vi "Keithley 2200 Series Execute a List.vi"() -> ()   [LabVIEW 2021]
doc: "DESCRIPTION:\n\nIn this VI commands executed in a certain order to run the list file. \n\nINSTRUCTIONS:\n1. Enter the resource name.\n2. Configures the power supply for command List mode\n3. Recall operation , recall list file from memory \n4. Enter Non -volatile memory address, that the settings will be saved to. \n5. Enable output of the power supply.\n6. Set trigger command to run the list file.\n7. Run the VI.\n\nNOTES:\n\nNotice the order of the power supply component VIs in the block diagram. The first VI in a sequence is the power supply Initialize.vi, which provides a VISA session to the instrument driver. The last VI in a sequence must be the power supply Close.vi which closes the Visa session."
uses:
  <instrlib>/Keithley 2200 Series/Keithley 2200 Series.lvlib
panel:
  in  "Enable Output (T: Enable)":bool=TRUE
  in  "VISA resource name":refnum<visa-resource-name>
  in  "Memory Address(1)":dbl=1.0
  # "(c) Copyright 2012 Keithley Instruments Inc  ALL RIGHTS RESERVED."
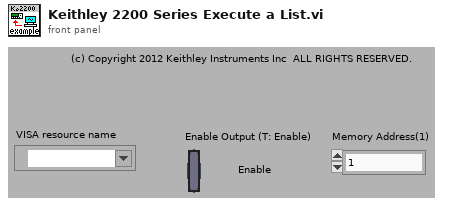
[diagram p1: front panel]
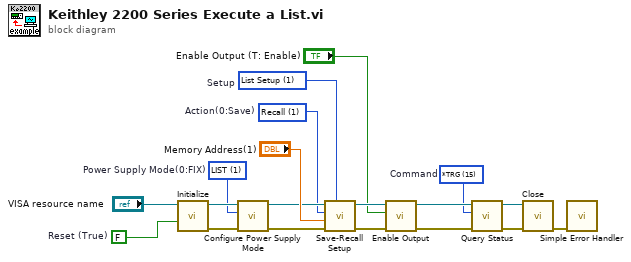
[diagram p0: block diagram]
diagram:
  w1 = u16 1 items=["Instrument Setup", "List Setup"]  # Setup
  w4 = u16 1 items=["Save", "Recall"]  # Action(0:Save)
  w12 = u16 15 items=["*CLS", "*ESE", "*ESE?", "*RST", "*SRE", "*SRE?", "*STB?", "*ESR?", "*IDN?", "*OPC", "*OPC?", "*PSC", "*PSC?", "*SAV", "*RCL", "*TRG", "System Address", "Output State", "Output-Timer", "Output-Timer-State", "Digital Input Port- State", "Digital Output Port- State"]  # Command
  w3 = u16 1 items=["FIX", "LIST", "Digital milliohm meter "]  # Power Supply Mode(0:FIX)
  w2 = FALSE items=["OFF", "ON", "OFF", "ON"]  # Reset (True)
  n1 = call <instrlib>:"Initialize.vi"("Reset (True)"=w2, "VISA resource name"="VISA resource name") -> ("error out"=w8:errorcluster, "VISA resource name out"=w9:refnum<visa-resource-name>)  [unwired: 3 in, 5 out]
  n2 = call <instrlib>:"Configure Power Supply Mode.vi"("error in (no error)"=w8, "Power Supply Mode (0:Fix)"=w3, "VISA resource name"=w9) -> ("error out"=w10:errorcluster, "VISA resource name out"=w11:refnum<visa-resource-name>)  [unwired: 7 out]
  n3 = call <instrlib>:"Save-Recall Setup.vi"("Setup(0:Instrument Setup)"=w1, "error in (no error)"=w10, "Memory Address(1)"="Memory Address(1)", "Action(0:Save)"=w4, "VISA resource name"=w11) -> ("error out"=w6:errorcluster, "VISA resource name out"=w7:refnum<visa-resource-name>)  [unwired: 5 out]
  n4 = call <instrlib>:"Enable Output.vi"("error in (no error)"=w6, "Enable Output (T: Enable)"="Enable Output (T: Enable)", "VISA resource name"=w7) -> ("error out"=w15:errorcluster, "VISA resource name out"=w16:refnum<visa-resource-name>)  [unwired: 7 out]
  n5 = call <instrlib>:"Query Status.vi"("error in (no error)"=w15, "Command (0:*CLS)"=w12, "VISA resource name"=w16) -> ("error out"=w13:errorcluster, "VISA resource name out"=w14:refnum<visa-resource-name>)  [unwired: 2 in, 5 out]
  n6 = call <instrlib>:"Close.vi"("error in (no error)"=w13, "VISA resource name"=w14) -> ("error out"=w17:errorcluster)  [unwired: 9 out]
  n7 = call <vilib>:"Simple Error Handler.vi"("error in (no error)"=w17) -> ()  [unwired: 1 in, 8 out]
